vi "MW_Display_Py_Get_Frame_Dims.vi"(0 "session in":refnum<k35>, 5 "module path":path=path "D:/dev/Guy_Storage/Work/Cancun/MW_Display_Test/Magewell Capture/Capture_LV.py", 11 "error in":errorcluster) -> (4 "session out":refnum<k35>, 6 "module path out":path, 14 "Frame Dims":T1, 15 "error out":errorcluster)   [LabVIEW 2023]
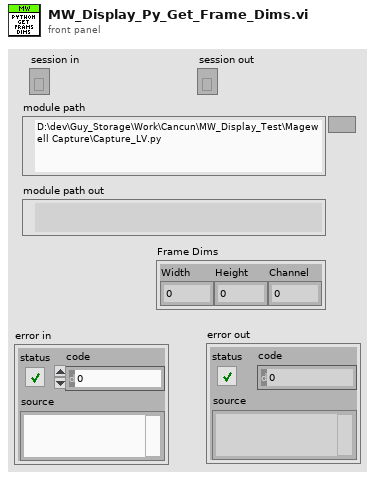
[diagram p1: front panel]
types:
  T1 = cluster{"Width":i32, "Height":i32, "Channel":i32}
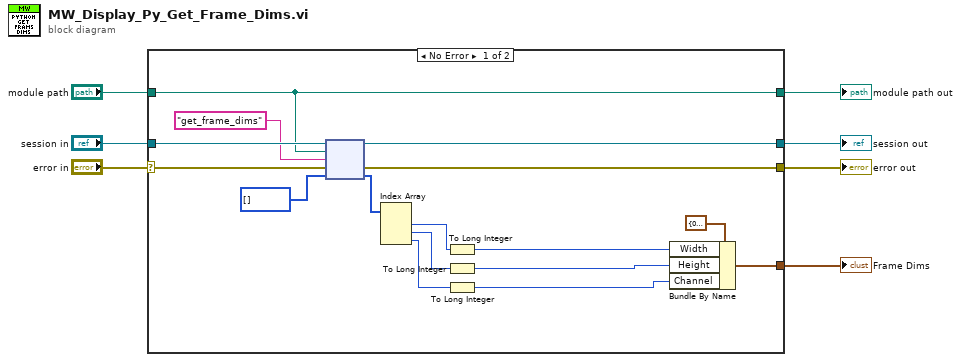
[diagram p0: block diagram]
diagram:
  n1 = case shown="No Error" "error in" {
    selector: "error in" -> [w20 w25]
    tunnel: "module path" -> [w18 w24]
    tunnel: "session in" -> [w23 w26]
    tunnel: [w22 w25] -> w3
    tunnel: [w21 w26] -> w5
    tunnel: [w18 w24] -> w2
    tunnel: [w8 _] -> w1
    frame No Error {
      n2 = node(w23, w18, "get_frame_dims" ("function name"), w20, i32[] []) -> (w21:refnum<k35>, w22:errorcluster, w16:i32[])  [unwired: 2 out]
      n3 = Index Array(array=w16) -> (element #1=w13:i32, element #2=w12:i32, element #3=w10:i32)  [unwired: 3 in]
      n4 = To Long Integer(number=w13) -> (32bit integer=w14:i32)
      n5 = To Long Integer(number=w12) -> (32bit integer=w11:i32)
      n6 = To Long Integer(number=w10) -> (32bit integer=w9:i32)
      n7 = Bundle By Name(cluster=T1 {"Width"=0, "Height"=0, "Channel"=0}, "Width"=w14, "Height"=w11, "Channel"=w9) -> (w8:T1)
    }
    frame Error {
    }
  }
  "session out" <- w5
  "error out" <- w3
  "module path out" <- w2
  "Frame Dims" <- w1
